vi "Mysql data reader scalar integer.vi"(8 "error in (no error)":errorcluster, 11 ".NET Refnum in":refnum<k24>) -> (0 "error out":errorcluster, 3 "GetString":i32)   [LabVIEW 2020, in "mysql.lvlib" / "mysql.lvclass"]
uses:
  mysql.lvclass
  MySql.Data
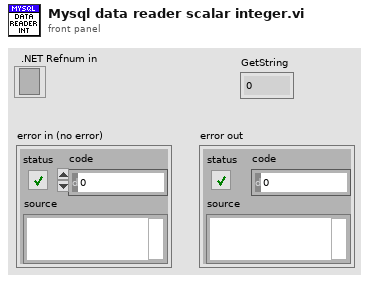
[diagram p1: front panel]
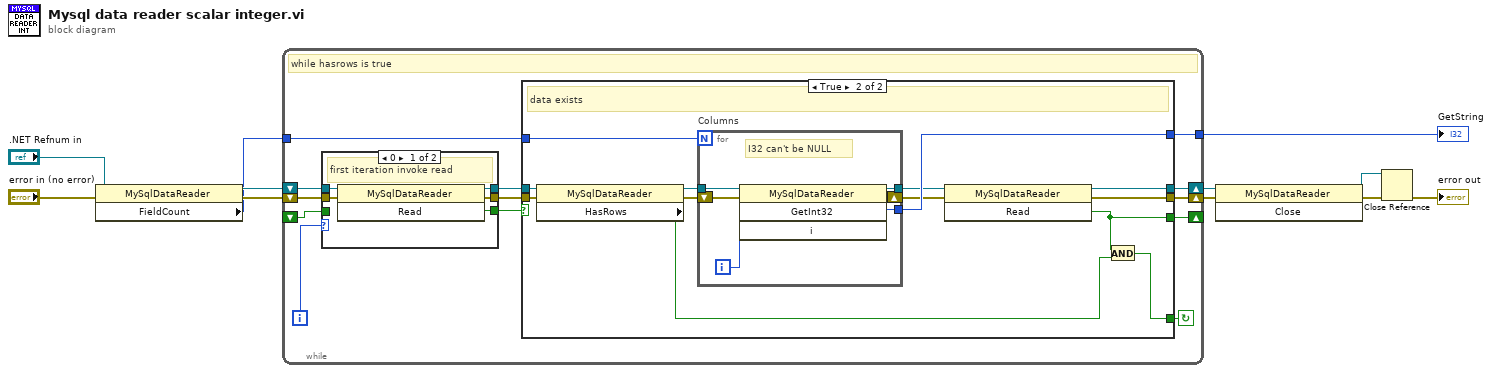
[diagram p0: block diagram]
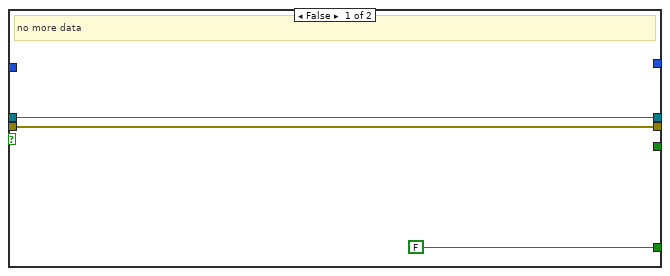
[diagram p3: hidden frame]
diagram:
  n1 = property class="MySqlDataReader"(reference=".NET Refnum in", error in="error in (no error)") -> (reference out=w7:refnum<k24>, error out=w6:errorcluster, "FieldCount"=w3:i32)
  n2 = while {
    tunnel: w3 -> [w24]
    tunnel: [w23] -> w4
    shift-right: [w21] -> w9
    shift-left: w6 -> [w17]
    shift-right: [w22] -> w8
    shift-left: w7 -> [w18]
    shift-right: [w19] -> _
    shift-left: _ -> [w16]
    i -> [w15]
    stop <- w20 continue-if-true
    # "while hasrows is true"
    n3 = case shown="0" w15 {
      tunnel: w17 -> [w29 w31]
      tunnel: [w28 w31] -> w14
      tunnel: w18 -> [w27 w32]
      tunnel: [w26 w32] -> w12
      tunnel: [w25 w30] -> w13
      tunnel: w16 -> [_ w30]
      frame 0 {
        # "first iteration invoke read"
        n4 = invoke class="MySqlDataReader" method="Read"(reference=w27, error in=w29) -> (reference out=w26:refnum<k24>, error out=w28:errorcluster, "Read"=w25:bool)  [unwired: 1 in]
      }
      frame 1.., Default {
        # "read after for other iterations"
      }
    }
    n5 = case shown="True" w13 {
      tunnel: w24 -> [_ w48]
      tunnel: [_ w47] -> w23
      tunnel: w14 -> [w34 w46]
      tunnel: w12 -> [w35 w45]
      tunnel: [w35 w38] -> w22
      tunnel: [w34 w39] -> w21
      tunnel: [FALSE ("HasRows") w41] -> w20
      tunnel: [_ w36] -> w19
      frame False {
        # "no more data"
      }
      frame True {
        # "data exists"
        n6 = property class="MySqlDataReader"(reference=w45, error in=w46) -> (reference out=w44:refnum<k24>, error out=w43:errorcluster, "HasRows"=w42:bool)
        n7 = for "Columns" {
          N: w48 -> [_]
          tunnel: w44 -> [w49]
          shift-right: [w54] -> w40
          shift-left: w43 -> [w50]
          tunnel: [w53] -> w47
          tunnel: [w52] -> w37
          i -> [w51]
          # "I32 can't be NULL"
          n8 = invoke class="MySqlDataReader" method="GetInt32"(reference=w49, error in=w50, "i"=w51) -> (reference out=w52:refnum<k24>, error out=w54:errorcluster, "GetInt32"=w53:i32)  [unwired: 1 in, 1 out]
        }
        n9 = invoke class="MySqlDataReader" method="Read"(reference=w37, error in=w40) -> (reference out=w38:refnum<k24>, error out=w39:errorcluster, "Read"=w36:bool)  [unwired: 1 in]
        n10 = And(x=w36, y=w42) -> (x .and. y?=w41:bool)
      }
    }
  }
  "GetString" <- w4
  n11 = invoke class="MySqlDataReader" method="Close"(reference=w8, error in=w9) -> (reference out=w11:refnum<k24>, error out=w10:errorcluster)  [unwired: 1 in, 1 out]
  n12 = Close Reference(reference=w11, error in (no error)=w10) -> (error out=→"error out":errorcluster)
